vi "MotionMagicConfig.vi"() -> ()   [LabVIEW 2018]
uses:
  2019_Robot_Code/Subsystems/Drive/driveShifterEnum.ctl
panel:
  in  "F":dbl=0.13335
  in  "D":dbl
  in  "I":dbl
  in  "P":dbl=0.0025
  in  "Acceleration":i32=10
  in  "Cruise Velocity":i32=6
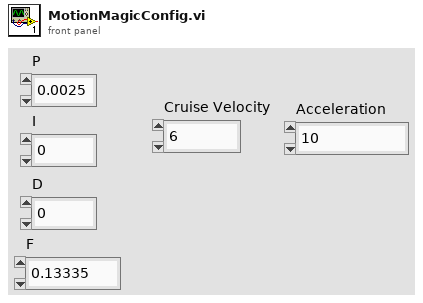
[diagram p1: front panel]
types:
  T1 = typedef "driveShifterEnum.ctl" = enum16{"Low", "High"}
  T2 = enum16{"Inches -> Sensor Units", "Sensor Units -> Inches"}
  T3 = typedef "WPI_MotorControlDeviceRef.ctl" = cluster{"DeviceStatus":errorcluster, "Type":T4, "PWM":cluster{"PWM Channel":T5, "DeadBand":T6}, "CAN":cluster{"Device Number":u8, "SetOutput VI Ref":variant, "GetOutput VI Ref":variant, "Enable VI Ref":variant, "Disable VI Ref":variant, "Data":variant}, "Invert":bool, "DIO PWM":cluster{"PWM \"Enable\" Channel":T5, "DIOChannel":T7, "PWM Rate":dbl}}
  T4 = typedef "WPI_MotorControlType.ctl" = enum16{"PWM", "CAN", "DIO PWM"}
  T5 = typedef "FPGA_DIOPWMChannel.ctl" = enum8{"PWM 0", "PWM 1", "PWM 2", "PWM 3", "PWM 4", "PWM 5", "PWM 6", "PWM 7", "PWM 8", "PWM 9", "PWM MXP 0", "PWM MXP 1", "PWM MXP 2", "PWM MXP 3", "PWM MXP 4", "PWM MXP 5", "PWM MXP 6", "PWM MXP 7", "PWM MXP 8", "PWM MXP 9", "Invalid"}
  T6 = typedef "WPI_PWMDeadband.ctl" = cluster{"Name":string, "maxPositivePwm":i32, "minPositivePwm":i32, "centerPwm":i32, "maxNegativePwm":i32, "minNegativePwm":i32, "angularRange":u16}
  T7 = typedef "FPGA_DIOChannel.ctl" = enum8{"DIO 0", "DIO 1", "DIO 2", "DIO 3", "DIO 4", "DIO 5", "DIO 6", "DIO 7", "DIO 8", "DIO 9", "DIO MXP 0", "DIO MXP 1", "DIO MXP 2", "DIO MXP 3", "DIO MXP 4", "DIO MXP 5", "DIO MXP 6", "DIO MXP 7", "DIO MXP 8", "DIO MXP 9", "DIO MXP 10", "DIO MXP 11", "DIO MXP 12", "DIO MXP 13", "DIO MXP 14", "DIO MXP 15", "SPI Port CS1", "SPI Port CS2", "SPI Port CS3", "SPI Port MISO", "SPI Port MOSI", "Invalid"}
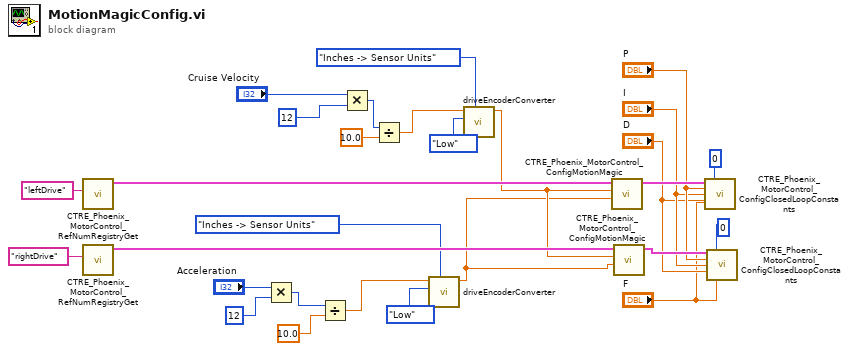
[diagram p0: block diagram]
diagram:
  n1 = call <vilib>:"CTRE_Phoenix_MotorControl_RefNumRegistryGet.vi"("refnum name"="leftDrive") -> ("PhoenixMotorControlDevRef"=w28:T3)  [unwired: 9 in, 1 out]
  n2 = call <vilib>:"CTRE_Phoenix_MotorControl_RefNumRegistryGet.vi"("refnum name"="rightDrive") -> ("PhoenixMotorControlDevRef"=w27:T3)  [unwired: 9 in, 1 out]
  n3 = Multiply(x="Acceleration", y=12) -> (x*y=w4:i32)
  n4 = Divide(x=w4, y=10.0) -> (x/y=w2:dbl)
  n5 = Multiply(x="Cruise Velocity", y=12) -> (x*y=w12:i32)
  n6 = Divide(x=w12, y=10.0) -> (x/y=w11:dbl)
  n7 = call "driveEncoderConverter.vi"("Conversion Direction"=T2."Inches -> Sensor Units", "Gear Setting"=driveShifterEnum."Low", "Input"=w2) -> ("Output"=w1:dbl)  [unwired: 8 in]
  n8 = call "driveEncoderConverter.vi"("Conversion Direction"=T2."Inches -> Sensor Units", "Gear Setting"=driveShifterEnum."Low", "Input"=w11) -> ("Output"=w9:dbl)  [unwired: 8 in]
  n9 = call <vilib>:"CTRE_Phoenix_MotorControl_ConfigMotionMagic.vi"("Acceleration"=w1, "Cruise Velocity"=w9, "PhoenixMotorControlDevRef"=w28) -> ("PhoenixMotorControlDevRef"=w24:T3)  [unwired: 7 in, 1 out]
  n10 = call <vilib>:"CTRE_Phoenix_MotorControl_ConfigMotionMagic.vi"("Acceleration"=w1, "Cruise Velocity"=w9, "PhoenixMotorControlDevRef"=w27) -> ("PhoenixMotorControlDevRef"=w23:T3)  [unwired: 7 in, 1 out]
  n11 = call <vilib>:"CTRE_Phoenix_MotorControl_ConfigClosedLoopConstants.vi"("PhoenixMotorControlDevRef"=w24, "slotIdx"=0, "P"="P", "I"="I", "D"="D", "F"="F") -> ()  [unwired: 8 in, 2 out]
  n12 = call <vilib>:"CTRE_Phoenix_MotorControl_ConfigClosedLoopConstants.vi"("PhoenixMotorControlDevRef"=w23, "slotIdx"=0, "P"="P", "I"="I", "D"="D", "F"="F") -> ()  [unwired: 8 in, 2 out]
